vi "lvw proje.vi"() -> ()   [LabVIEW 2017]
uses:
  <vilib>/MakerHub/LINX/Private/Type Defs/Thumbstick Data.ctl
  <vilib>/MakerHub/LINX/Public/Utilities/Open Serial.vi
  <vilib>/MakerHub/LINX/LMH-LINX.lvlib
panel:
  in  "stop":bool
  out "XY Graph":cluster{dbl[], dbl[]}(graph)
  in  "Thumbstick Configuration":T1
  in  "Serial Port":refnum<visa-resource-name>="N/A"
  out "Thumbstick Data":T2
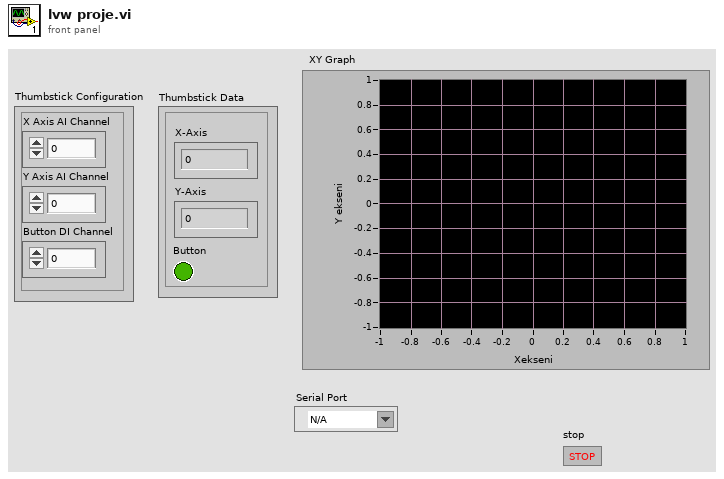
[diagram p1: front panel]
types:
  T1 = cluster{"X Axis AI Channel":u8, "Y Axis AI Channel":u8, "Button DI Channel":u8}
  T2 = typedef "LMH-LINX.lvlib/Thumbstick Data.ctl" = cluster{"X-Axis":dbl, "Y-Axis":dbl, "Button":bool}
  T3 = typedef "LMH-LINX.lvlib/LINX Ref.ctl" = cluster{"IO":T4, "Interface":T5, "LINX Device Config":T6}
  T4 = typedef "LMH-LINX.lvlib/Platform.ctl" = enum16{"Remote", "Local"}
  T5 = typedef "LMH-LINX.lvlib/Interface.ctl" = enum16{"Serial", "TCP"}
  T6 = typedef "LMH-LINX.lvlib/Device.lvlib/LINX Device Config.ctl" = cluster{"Interface":T5, "COM Port":refnum<visa-resource-name>, "TCP Configuration":T7, "Device Family":u8, "Device ID":u8, "Device Name":string, "TCP Ref":refnum<k5>, "Channels":T8}
  T7 = typedef "LMH-LINX.lvlib/Device.lvlib/TCP Config.ctl" = cluster{"IP Address":string, "Port":u16}
  T8 = typedef "LMH-LINX.lvlib/Channels.ctl" = cluster{"DI":u8[], "DO":u8[], "AI":u8[], "AO":u8[], "PWM":u8[], "QE":u8[], "UART":u8[], "I2C 2":u8[], "SPI":u8[], "CAN":u8[], "Servo":u8[], "AI Ref (V)":dbl, "AI Resolution (Bits)":u8, "AO Ref (V)":dbl, "AO Resolution (Bits)":u8}
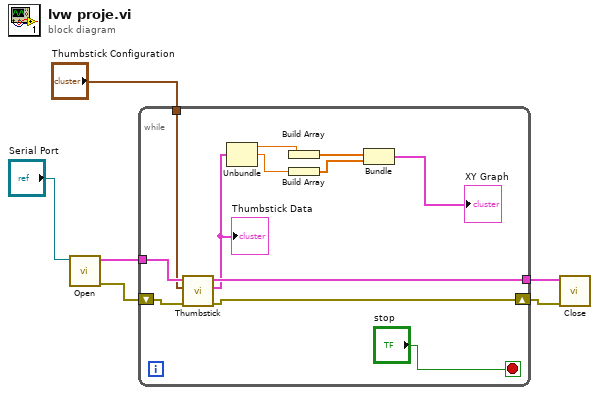
[diagram p0: block diagram]
diagram:
  n1 = call-poly <vilib>:"Open.vi"("Serial Port"="Serial Port") -> ("Error Out"=w2:errorcluster, "LINX Resource"=w6:T3)  [unwired: 8 in, 1 out]
  n2 = while {
    tunnel: w6 -> [w18]
    tunnel: [w17] -> w5
    tunnel: "Thumbstick Configuration" -> [w13]
    shift-right: [w9] -> w1
    shift-left: w2 -> [w10]
    stop <- "stop" stop-if-true
    n3 = call <vilib>:"Thumbstick.vi"("Error In"=w10, "Thumbstick Configuration"=w13, "LINX Resource"=w18) -> ("Error Out"=w9:errorcluster, "Thumbstick Data"=w16:T2, "LINX Resource"=w17:T3)  [unwired: 6 in]
    "Thumbstick Data" <- w16
    n4 = Unbundle(w16) -> ("X-Axis"=w15:dbl, "Y-Axis"=w14:dbl)  [unwired: 1 out]
    n5 = Build Array(w15) -> (w12:dbl[])
    n6 = Build Array(w14) -> (w11:dbl[])
    n7 = Bundle(w12, w11) -> (→"XY Graph":cluster{dbl[], dbl[]})  [unwired: 1 in]
  }
  n8 = call <vilib>:"Close.vi"("Error In"=w1, "LINX Resource"=w5) -> ()  [unwired: 9 in, 1 out]
